vi "Dropdown - PreLoops.vi"() -> (4 "Dropdown Bundle":T2, 15 "Error Out":errorcluster)   [LabVIEW 2013]
uses:
  <vilib>/Utility/miscctls.llb/LVRowAndColumnTypeDef.ctl
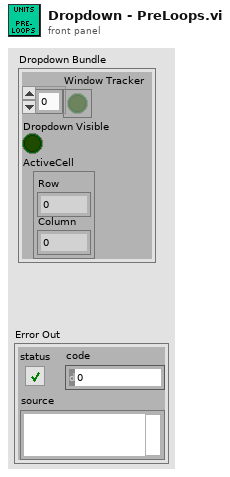
[diagram p1: front panel]
types:
  T1 = typedef "LVRowAndColumnTypeDef.ctl" = cluster{"Row":i32, "Column":i32}
  T2 = cluster{"Window Tracker":bool[], "Dropdown Visible":bool, "ActiveCell":T1}
  T3 = enum16{"Set Abbreviations", "Set Engine Mode", "Set Enum Position", "Get Abbreviation", "Write Abbreviation", "Read Enum Position", "Read Engine Mode", "Read Abbreviations", "Engine Started", "Check Engine", "Init Global", "Set Cursor", "Read Cursor"}
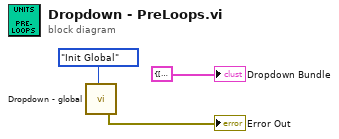
[diagram p0: block diagram]
diagram:
  n1 = call "Dropdown - global.vi"("Global Mode"=T3."Init Global") -> ("Error Out"=→"Error Out":errorcluster)  [unwired: 10 in, 8 out]
  "Dropdown Bundle" <- T2 {"Window Tracker"=[], "Dropdown Visible"=FALSE, "ActiveCell"={"Row"=0, "Column"=0}} ("Dropdown Bundle")
